vi "Render Thrust Dots.vi"(7 "Renderer":refnum<class "Renderer.lvclass">, 8 "error in (no error)":errorcluster, 10 "Camera":refnum<class "Camera.lvclass">, 11 "Ship in":refnum<class "Ship.lvclass">) -> (0 "error out":errorcluster)   [LabVIEW 2021, in "Ship.lvclass"]
uses:
  Ship.lvclass
  Camera/Camera.lvclass
  Renderer/Renderer.lvclass
  Ship.lvclass/Ship.ctl
  Thrust Dot/Thrust Dot.lvclass
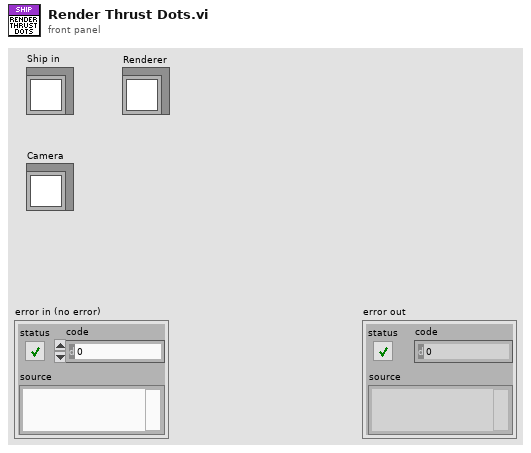
[diagram p1: front panel]
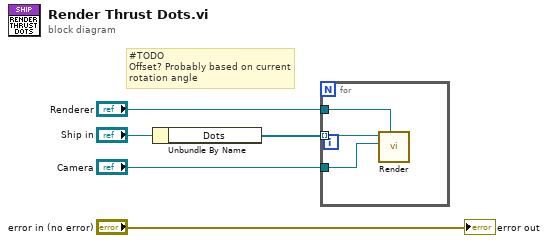
[diagram p0: block diagram]
diagram:
  # "#TODO\nOffset? Probably based on current rotation angle"
  n1 = Unbundle By Name("Ship in") -> ("Dots"=w4:refnum<class "Thrust Dot.lvclass">[])
  n2 = for {
    tunnel: w4 -> [w8] mode=indexing
    tunnel: "Camera" -> [w7]
    tunnel: "Renderer" -> [w6]
    n3 = call "Render.vi"("Renderer"=w6, "Camera"=w7, "Thrust Dot in"=w8) -> ()  [unwired: 9 in]
  }
  "error out" <- "error in (no error)"
